vi "CloseGripper.vi"(8 "error in (no error)":errorcluster caption="Fehler (Eingang, kein Fehler)", 11 "Moveo Eingang":refnum<class "Moveo.lvclass">) -> (0 "error out":errorcluster caption="Fehler (Ausgang)", 3 "Moveo Ausgang":refnum<class "Moveo.lvclass">)   [LabVIEW 2019, in "Moveo.lvclass"]
uses:
  Moveo.lvclass
  Moveo.lvclass/Moveo.ctl
  MoveoSerialClass/MoveoSerial.lvclass
panel:
  in  "Gripper":u8=100
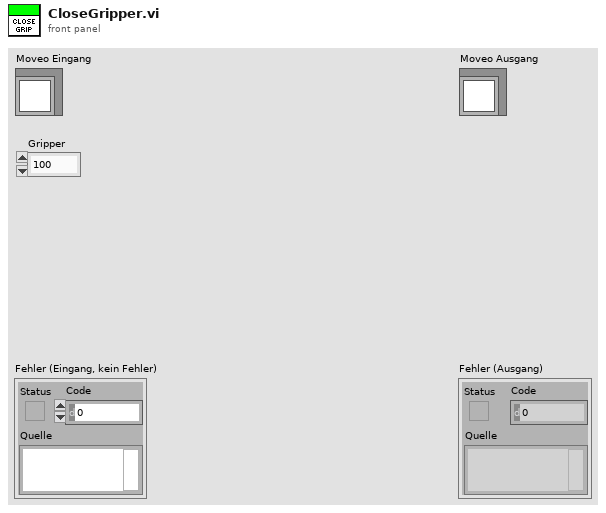
[diagram p1: front panel]
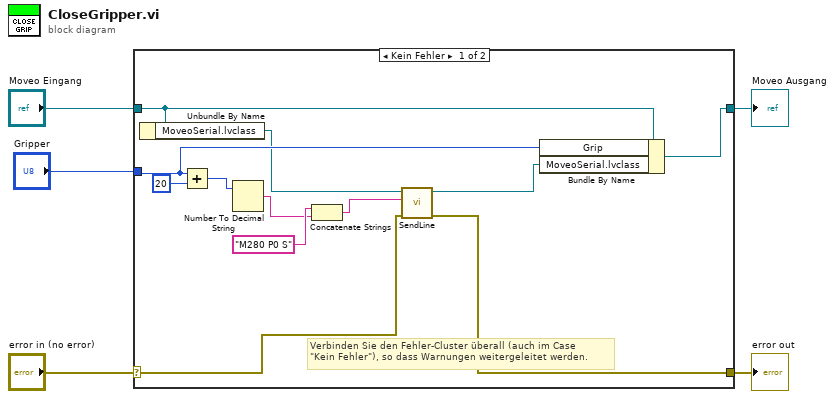
[diagram p0: block diagram]
diagram:
  n1 = case shown="Kein Fehler" "error in (no error)" {
    selector: "error in (no error)" -> [w7 w19]
    tunnel: [w6 w19] -> w4
    tunnel: [w16 w18] -> w2
    tunnel: "Moveo Eingang" -> [w10 w18]
    tunnel: "Gripper" -> [w15 _]
    frame No Error {
      # "Verbinden Sie den Fehler-Cluster überall (auch im Case\n\"Kein Fehler\"), so dass Warnungen weitergeleitet werden."
      n2 = Unbundle By Name(w10) -> ("MoveoSerial.lvclass"=w9:refnum<class "MoveoSerial.lvclass">)
      n3 = Add(x=w15, y=u8 20) -> (x+y=w14:u8)
      n4 = Number To Decimal String(number=w14) -> (decimal integer string=w12:string)  [unwired: 1 in]
      n5 = Concatenate Strings("M280 P0 S", w12) -> (w11:string)
      n6 = call-dynamic "SendLine.vi"("error in (no error)"=w7, "SendString"=w11, "MoveoSerial Eingang"=w9) -> ("error out"=w6:errorcluster, "MoveoSerial Ausgang"=w8:refnum<class "MoveoSerial.lvclass">)  [unwired: 7 in]
      n7 = Bundle By Name(cluster=w10, "Grip"=w15, "MoveoSerial.lvclass"=w8) -> (w16:refnum<class "Moveo.lvclass">)
    }
    frame Error {
    }
  }
  "error out" <- w4
  "Moveo Ausgang" <- w2
